vi "Write Logging Enabled.vi"(8 "error in (no error)":errorcluster, 10 "LoggingEnabled":bool, 11 "Engine in":refnum<class "Engine.lvclass">) -> (0 "error out":errorcluster, 3 "Engine out":refnum<class "Engine.lvclass">)   [LabVIEW 2023, in "Engine.lvlib" / "Engine.lvclass"]
doc: "Update the Logging Enabled Status Control"
uses:
  Library/Engine.lvclass
  Library/Engine.lvclass/Engine.ctl
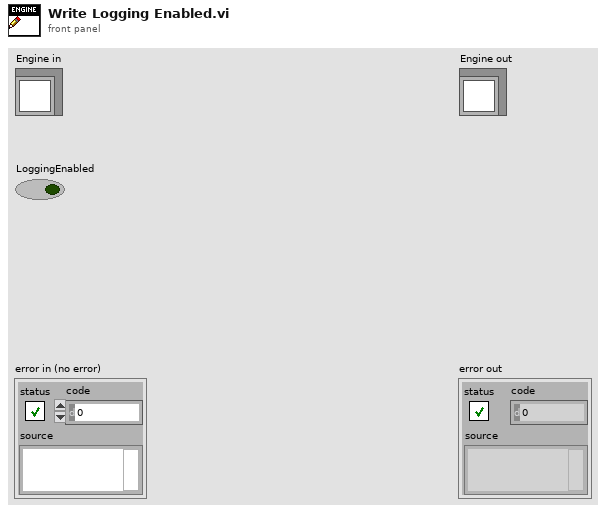
[diagram p1: front panel]
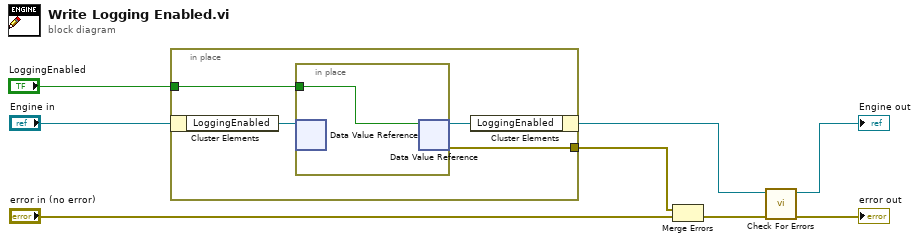
[diagram p0: block diagram]
diagram:
  n1 = in-place {
    in-place-border: "LoggingEnabled" -> [w11]
    in-place-border: [w9] -> w6
    n2 = in-place-cluster #1("Engine in") -> ("LoggingEnabled"=w12:refnum<data-value>)
    n3 = in-place {
      in-place-border: w11 -> [w13]
      n4 = in-place-dvr #2(w12) -> ()  [unwired: 2 out]
      n5 = in-place-dvr #2(w13) -> (w10:refnum<data-value>, w9:errorcluster)
    }
    n6 = in-place-cluster #1("LoggingEnabled"=w10) -> (w2:refnum<class "Engine.lvclass">)
  }
  n7 = Merge Errors(w6, "error in (no error)") -> (w4:errorcluster)
  n8 = call "Check For Errors.vi"("error in"=w4, "Engine in"=w2) -> ("error out"=→"error out":errorcluster, "Engine out"=→"Engine out":refnum<class "Engine.lvclass">)  [unwired: 8 in]
